vi "生成板卡编号.vi"() -> (2 "bCreate":bool)   [LabVIEW 2010]
uses:
  全局量/试验配置信息.vi
panel:
  out "temp":u64
  in  "temp":u64[](array[numeric])
  out "条形码":u64 step=1
  in  "btn_生成条形码":bool
  in  "btn_返回":bool
  in  "btn_打印":bool
  in  "板卡序号":u64 step=1
  in  "板卡类型":u64 max=99 step=1
  in  "软件版本号":u64 max=999 step=1
  in  "板卡大类":u64 min=1 max=9 step=1
  # "条 形 码 界 面"
  # "板卡大类："
  # "板卡类型："
  # "软件版本："
  # "板卡序号："
  # "板卡编号："
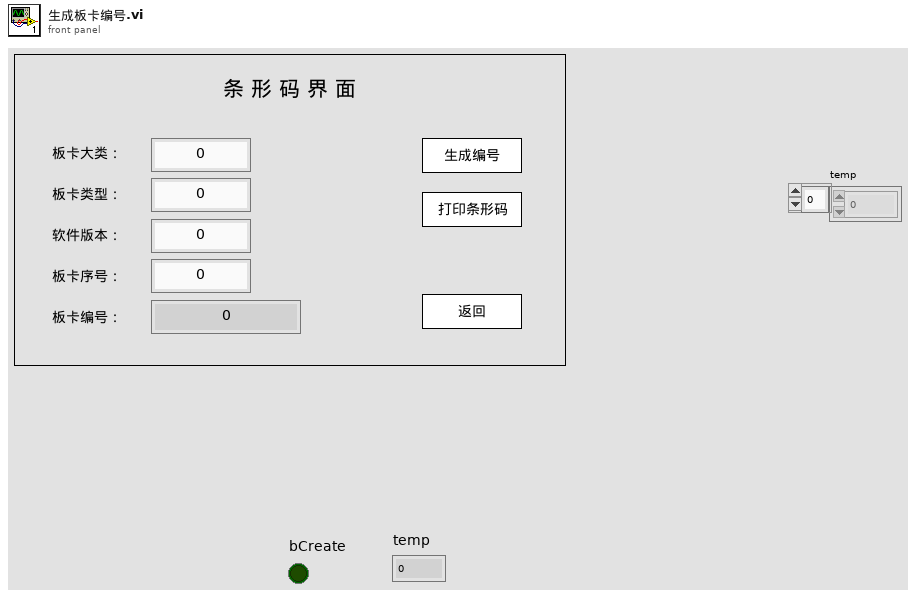
[diagram p1: front panel]
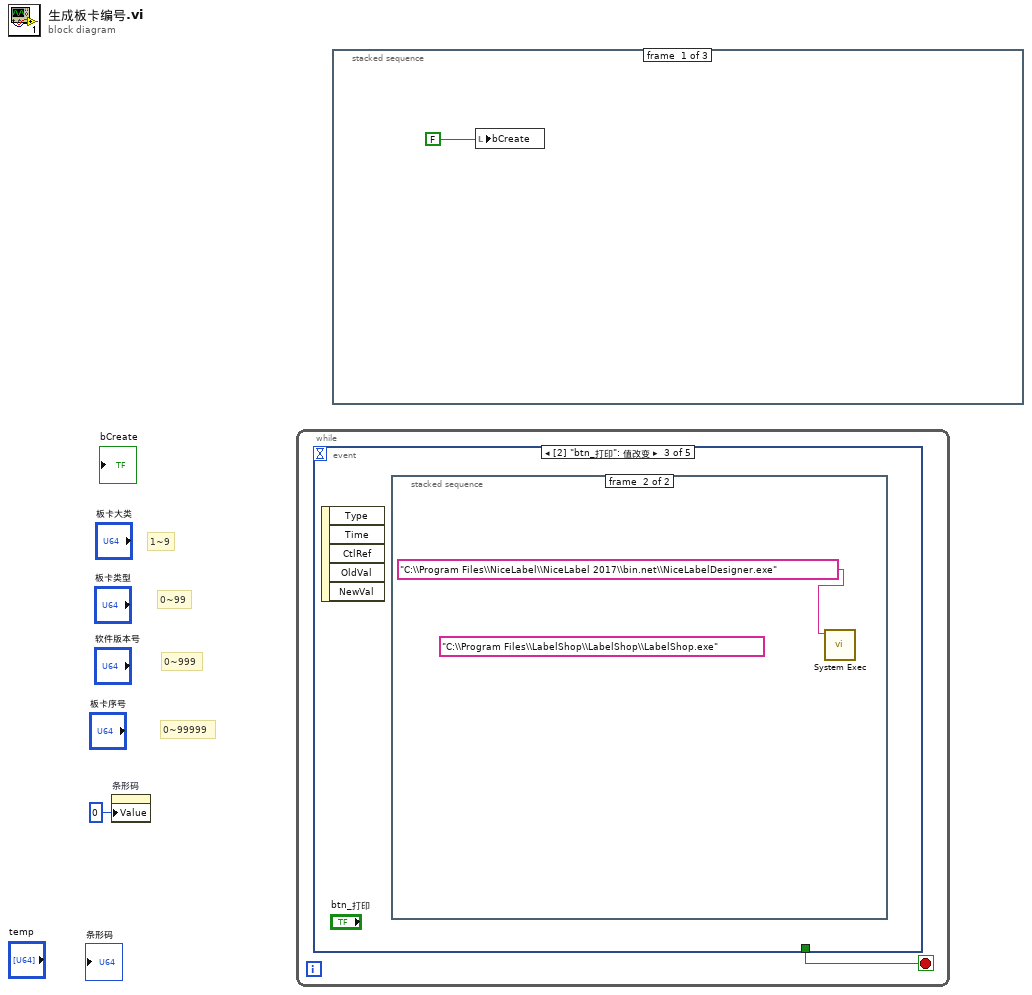
[diagram p0: block diagram]
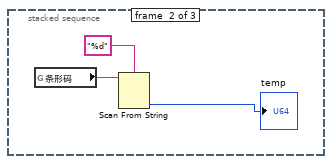
[diagram p2: hidden frame]
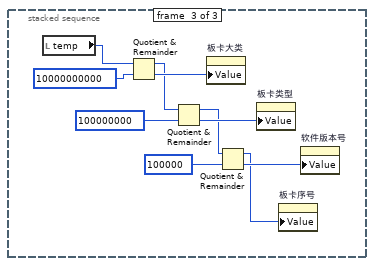
[diagram p3: hidden frame]
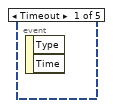
[diagram p4: hidden frame]
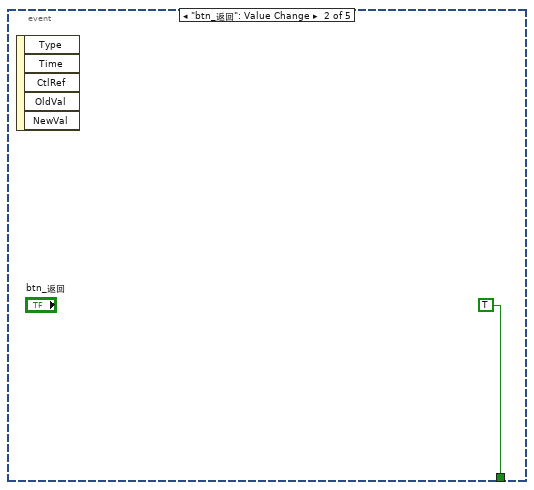
[diagram p5: hidden frame]
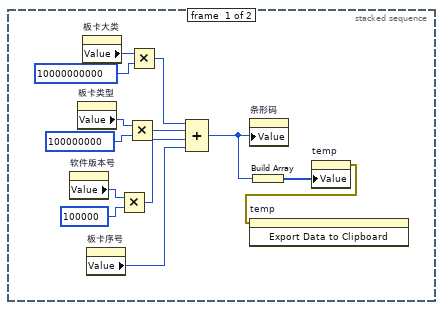
[diagram p6: hidden frame]
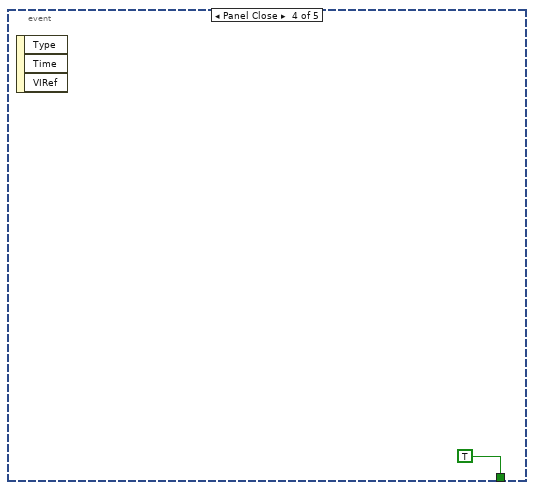
[diagram p7: hidden frame]
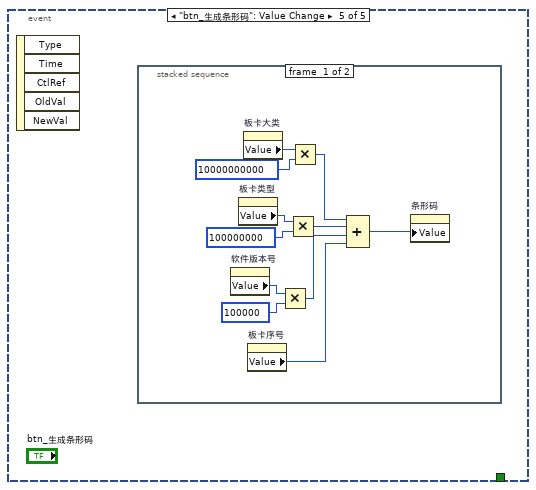
[diagram p8: hidden frame]
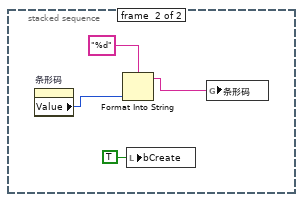
[diagram p9: hidden frame]
diagram:
  # "0~99999"
  # "0~999"
  # "0~99"
  # "1~9"
  n1 = property on="条形码" class="DigNum (严格)"("Value"=u64 0 ("条形码")) -> ()  [unwired: 2 in, 2 out]
  n2 = while {
    stop <- w2 stop-if-true
    n3 = event shown="[2] \"btn_打印\": 值改变" {
      selector: _ -> [_ _ _ _ _]
      dyn-events: _ -> [_ _ _ _ _]
      timeout: _ -> [_ _ _ _ _]
      tunnel: [_ TRUE _ TRUE _] -> w2
      event Timeout {
        n4 = event-data() -> ()  [unwired: 1 in, 2 out]
      }
      event "btn_返回": Value Change {
        n5 = event-data() -> ()  [unwired: 1 in, 5 out]
      }
      event "btn_打印": Value Change {
        n6 = event-data() -> ()  [unwired: 1 in, 5 out]
        n7 = stacked-sequence {
          frame #0 {
            n8 = property on="软件版本号" class="DigNum (严格)"() -> ("Value"=w12:u64)  [unwired: 2 in, 2 out]
            n9 = property on="板卡类型" class="DigNum (严格)"() -> ("Value"=w14:u64)  [unwired: 2 in, 2 out]
            n10 = property on="板卡大类" class="DigNum (严格)"() -> ("Value"=w16:u64)  [unwired: 2 in, 2 out]
            n11 = property on="板卡序号" class="DigNum (严格)"() -> ("Value"=w7:u64)  [unwired: 2 in, 2 out]
            n12 = Multiply(x=w12, y=u64 100000) -> (x*y=w8:u64)
            n13 = Multiply(x=w14, y=u64 100000000) -> (x*y=w9:u64)
            n14 = Multiply(x=w16, y=u64 10000000000) -> (x*y=w10:u64)
            n15 = Compound Arithmetic op=ADD(w10, w9, w8, w7) -> (w6:u64)
            n16 = property on="条形码" class="DigNum (严格)"("Value"=w6) -> ()  [unwired: 2 in, 2 out]
            n17 = Build Array(w6) -> (w5:u64[])
            n18 = property on="temp" class="Arr (严格)"("Value"=w5) -> (error out=w4:errorcluster)  [unwired: 2 in, 1 out]
            n19 = invoke on="temp" class="Arr (严格)" method="Export Data to Clipboard"(error in=w4) -> ()  [unwired: 2 in, 3 out]
          }
          frame #1 {
            (unwired) "C:\\Program Files\\LabelShop\\LabelShop\\LabelShop.exe"
            n20 = call <vilib>:"System Exec.vi"("command line"="C:\\Program Files\\NiceLabel\\NiceLabel 2017\\bin.net\\NiceLabelDesigner.exe") -> ()  [unwired: 7 in, 4 out]
          }
        }
      }
      event Panel Close {
        n21 = event-data() -> ()  [unwired: 1 in, 3 out]
      }
      event "btn_生成条形码": Value Change {
        n22 = event-data() -> ()  [unwired: 1 in, 5 out]
        n23 = stacked-sequence {
          frame #0 {
            n24 = property on="软件版本号" class="DigNum (严格)"() -> ("Value"=w25:u64)  [unwired: 2 in, 2 out]
            n25 = property on="板卡类型" class="DigNum (严格)"() -> ("Value"=w27:u64)  [unwired: 2 in, 2 out]
            n26 = property on="板卡大类" class="DigNum (严格)"() -> ("Value"=w29:u64)  [unwired: 2 in, 2 out]
            n27 = property on="板卡序号" class="DigNum (严格)"() -> ("Value"=w20:u64)  [unwired: 2 in, 2 out]
            n28 = Multiply(x=w25, y=u64 100000) -> (x*y=w21:u64)
            n29 = Multiply(x=w27, y=u64 100000000) -> (x*y=w22:u64)
            n30 = Multiply(x=w29, y=u64 10000000000) -> (x*y=w23:u64)
            n31 = Compound Arithmetic op=ADD(w23, w22, w21, w20) -> (w19:u64)
            n32 = property on="条形码" class="DigNum (严格)"("Value"=w19) -> ()  [unwired: 2 in, 2 out]
          }
          frame #1 {
            n33 = property on="条形码" class="DigNum (严格)"() -> ("Value"=w33:u64)  [unwired: 2 in, 2 out]
            n34 = Format Into String(format string="%d" ("格式字符串"), w33) -> (resulting string=w32:string)  [unwired: 2 in, 1 out]
            n35 = local write "bCreate"(TRUE ("bCreate")) -> ()
            n36 = global write "试验配置信息.vi" "条形码"(w32) -> ()
          }
        }
      }
    }
  }
  n37 = stacked-sequence {
    frame #0 {
      n38 = local write "bCreate"(FALSE) -> ()
    }
    frame #1 {
      n39 = global read "试验配置信息.vi" "条形码"() -> (w37:string)
      n40 = Scan From String(format string="%d" ("格式字符串"), input string=w37) -> (output 1=→"temp":u64)  [unwired: 3 in, 3 out]
    }
    frame #2 {
      n41 = local read "temp"() -> (w47:u64)
      n42 = Quotient & Remainder(x=w47, y=u64 10000000000) -> (x-y*floor(x/y)=w44:u64, floor(x/y)=w45:u64)
      n43 = Quotient & Remainder(x=w44, y=u64 100000000) -> (x-y*floor(x/y)=w40:u64, floor(x/y)=w42:u64)
      n44 = property on="板卡大类" class="DigNum (严格)"("Value"=w45) -> ()  [unwired: 2 in, 2 out]
      n45 = Quotient & Remainder(x=w40, y=u64 100000) -> (x-y*floor(x/y)=w38:u64, floor(x/y)=w41:u64)
      n46 = property on="板卡类型" class="DigNum (严格)"("Value"=w42) -> ()  [unwired: 2 in, 2 out]
      n47 = property on="板卡序号" class="DigNum (严格)"("Value"=w38) -> ()  [unwired: 2 in, 2 out]
      n48 = property on="软件版本号" class="DigNum (严格)"("Value"=w41) -> ()  [unwired: 2 in, 2 out]
    }
  }
